vi "Encrypt.vi"(8 "error in (no error)":errorcluster, 10 "Plaintext":string, 11 "Cipher in":refnum<class "Cipher.lvclass">) -> (0 "error out":errorcluster, 2 "Cyphertext":string, 3 "Cipher out":refnum<class "Cipher.lvclass">)   [LabVIEW 2020, in "Cipher.lvclass"]
doc: "Override this VI to convert plaintext into an encrypted string. The parent class implementation returns the input string without modification."
uses:
  Cipher.lvclass
  Cipher.lvclass/Cipher.ctl
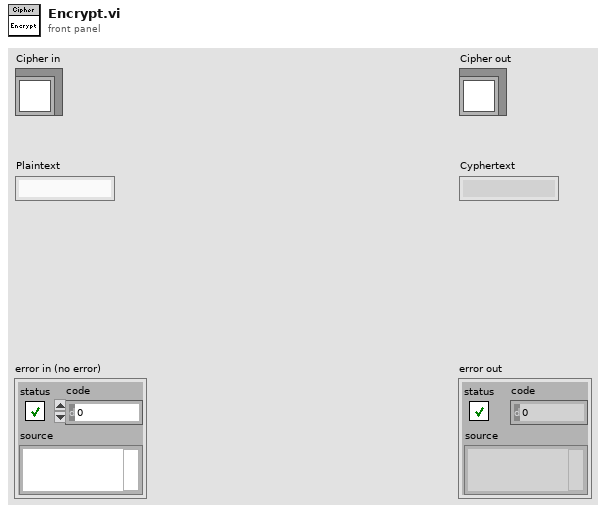
[diagram p1: front panel]
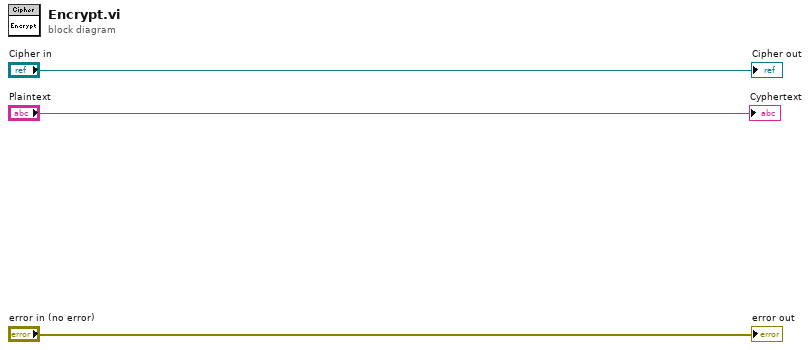
[diagram p0: block diagram]
diagram:
  "error out" <- "error in (no error)"
  "Cipher out" <- "Cipher in"
  "Cyphertext" <- "Plaintext"
